vi "Send Data.vi"(7 "Data DVR":refnum<data-value>, 8 "Error In":errorcluster, 11 "Communication in":refnum<class "Communication.lvclass">) -> (0 "Error Out":errorcluster, 3 "Communication out":refnum<class "Communication.lvclass">)   [LabVIEW 2020, in "Communication.lvclass"]
doc: "The method is a over riding method to send data to the receiver class."
uses:
  Communication.lvclass
  Data/Data.lvclass
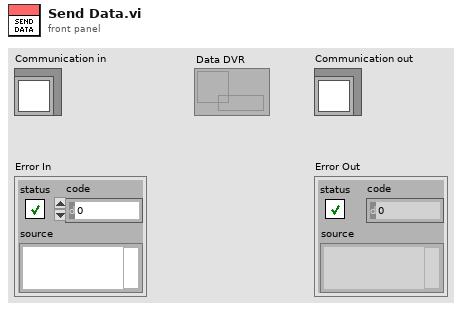
[diagram p1: front panel]
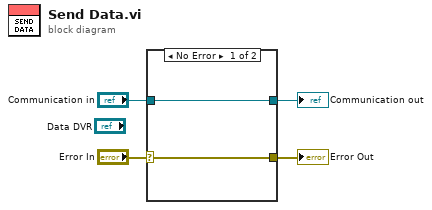
[diagram p0: block diagram]
diagram:
  n1 = case shown="No Error" "Error In" {
    selector: "Error In" -> [w5 w8]
    tunnel: [w5 w8] -> w3
    tunnel: [w6 w7] -> w1
    tunnel: "Communication in" -> [w6 w7]
    frame No Error {
    }
    frame Error {
    }
  }
  "Error Out" <- w3
  "Communication out" <- w1
